vi "ReportStatus.vi"(1 "Destination":T1={"Subsystem Id"=90, "Node Id"=1, "Component Id"=1}, 2 "Status":u8(ring)=2 items=["INIT", "READY", "STANDBY", "SHUTDOWN", "FAILURE", "EMERGENCY"], 3 "Source":T1={"Subsystem Id"=3, "Node Id"=1, "Component Id"=1}) -> (0 "Encoded JAUS Message":string)   [LabVIEW 2009]
uses:
  Support Files/Address.ctl
panel:
  in  "Reserved Field":u32
  in  "Command Code":string="@\u0002"
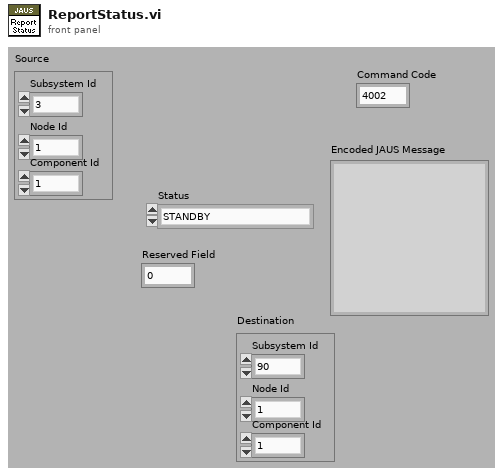
[diagram p1: front panel]
types:
  T1 = typedef "Address.ctl" = cluster{"Subsystem Id":u16, "Node Id":u8, "Component Id":u8}
  T2 = cluster{"unsigned byte array[0]":u8, "unsigned byte array[1]":u8}
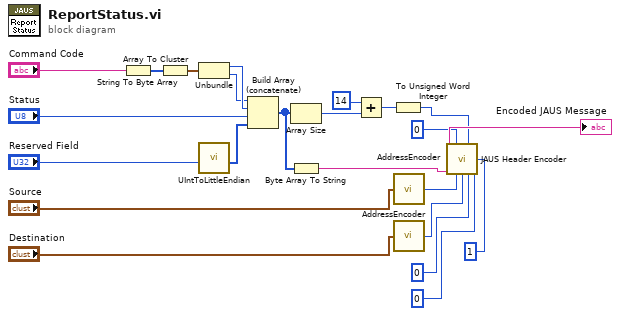
[diagram p0: block diagram]
diagram:
  n1 = String To Byte Array(string="Command Code") -> (unsigned byte array=w9:u8[])
  n2 = Array To Cluster(array=w9) -> (cluster=w8:T2)
  n3 = Unbundle(w8) -> ("unsigned byte array[0]"=w7:u8, "unsigned byte array[1]"=w6:u8)
  n4 = call "UIntToLittleEndian.vi"("Number"="Reserved Field") -> ("byte array"=w4:u8[])  [unwired: 10 in]
  n5 = Build Array (concatenate)(w6, w7, "Status", w4) -> (w13:u8[])
  n6 = Array Size(array=w13) -> (size(s)=w11:i32)
  n7 = Byte Array To String(unsigned byte array=w13) -> (string=w15:string)
  n8 = Add(x=14, y=w11) -> (x+y=w10:i32)
  n9 = To Unsigned Word Integer(number=w10) -> (unsigned 16bit integer=w1:u16)
  n10 = call "AddressEncoder.vi"("Address Cluster"="Source") -> ("Address"=w22:u32)
  n11 = call "AddressEncoder.vi"("Address Cluster"="Destination") -> ("Address"=w21:u32)
  n12 = call "JAUS Header Encoder.vi"("Message Type (0-5)"=u8 0, "Data Size (8-23)"=w1, "Priority(40-41)"=u8 1, "Payload"=w15, "Source ID (80-95)"=w22, "Destination ID (48-79)"=w21, "Data Flags (46-47)"=u8 0, "Ack/Nak (44-45)"=u8 0) -> ("Encoded JAUS Message"=→"Encoded JAUS Message":string)  [unwired: 7 in]
